vi "Test02_GPU_vs_CPU_Erode.vi"() -> ()   [LabVIEW 2018]
uses:
  <vilib>/vision/NI_Vision_Development_Module.lvlib
  <userlib>/_MGI/1D Array/MGI Average/MGI Average (SGL[]).vi
panel:
  out "Processor History":sgl(graph)
  in  "Stop CPU 2":bool
  out "CPU Average":sgl
  out "error out":errorcluster
  out "CPU Usage (%)":sgl(slide) scale=0.0..100.0
  in  "Time Target (s)":dbl=20.0
  in  "Erode radio":i32=1
  in  "Threshold max":i32=240
  in  "Threshold min":i32=70
  in  "Image Path":path=path "D:/UJI/TFG/TFG_Repositorio/Proyecto/img_to_erode_media.png"
  in  "Start":bool
  in  "Stop GPU":bool
  in  "Stop CPU":bool
  in  "Erode kernel":i32[][](array[numeric])=[[1, 1, 1], [1, 1, 1], [1, 1, 1]]
  out "Image Out CPU":T1(plugin-control)
  out "Image In":T1(plugin-control)
  out "Image Out GPU":T1(plugin-control)
  out "Processed Images":i32
  in  "Threshold range":cluster{"Lower value":sgl, "Upper value":sgl}={"Lower value"=70.0, "Upper value"=240.0} {"Upper value" format="%.2f"; "Lower value" format="%.2f"}
  out "Threhsold Time (ms)":dbl
  out "Erode Time (ms)":dbl
  out "Total Time (ms)":dbl
  out "Error out CPU":errorcluster
  in  "Error in":errorcluster caption="Error in CPU (no error)"
  out "error_cuda_free":i32
  out "error_gpu_to_cpu":i32
  out "error_cpu_to_gpu":i32
  out "Cuda Free Time (ms)":dbl
  out "Set IMG Param Time (ms)":dbl
  out "Total Time (ms)":dbl
  out "Copy to CPU Time (ms)":dbl
  out "Erode Time (ms)":dbl
  out "Threshold Time (ms)":dbl
  out "Copy to GPU Time (ms)":dbl
  out "Processed Images":i32
  out "Error out GPU":errorcluster
  in  "Error":errorcluster caption="Error in GPU (no error)"
  # "GPU CUDA -"
  # "ERODE - GPU vs CPU"
  # "GPU Time Results"
  # "Configuration"
  # "CPU Time Results"
  # "GPU Parameters"
  # "CPU Parameters"
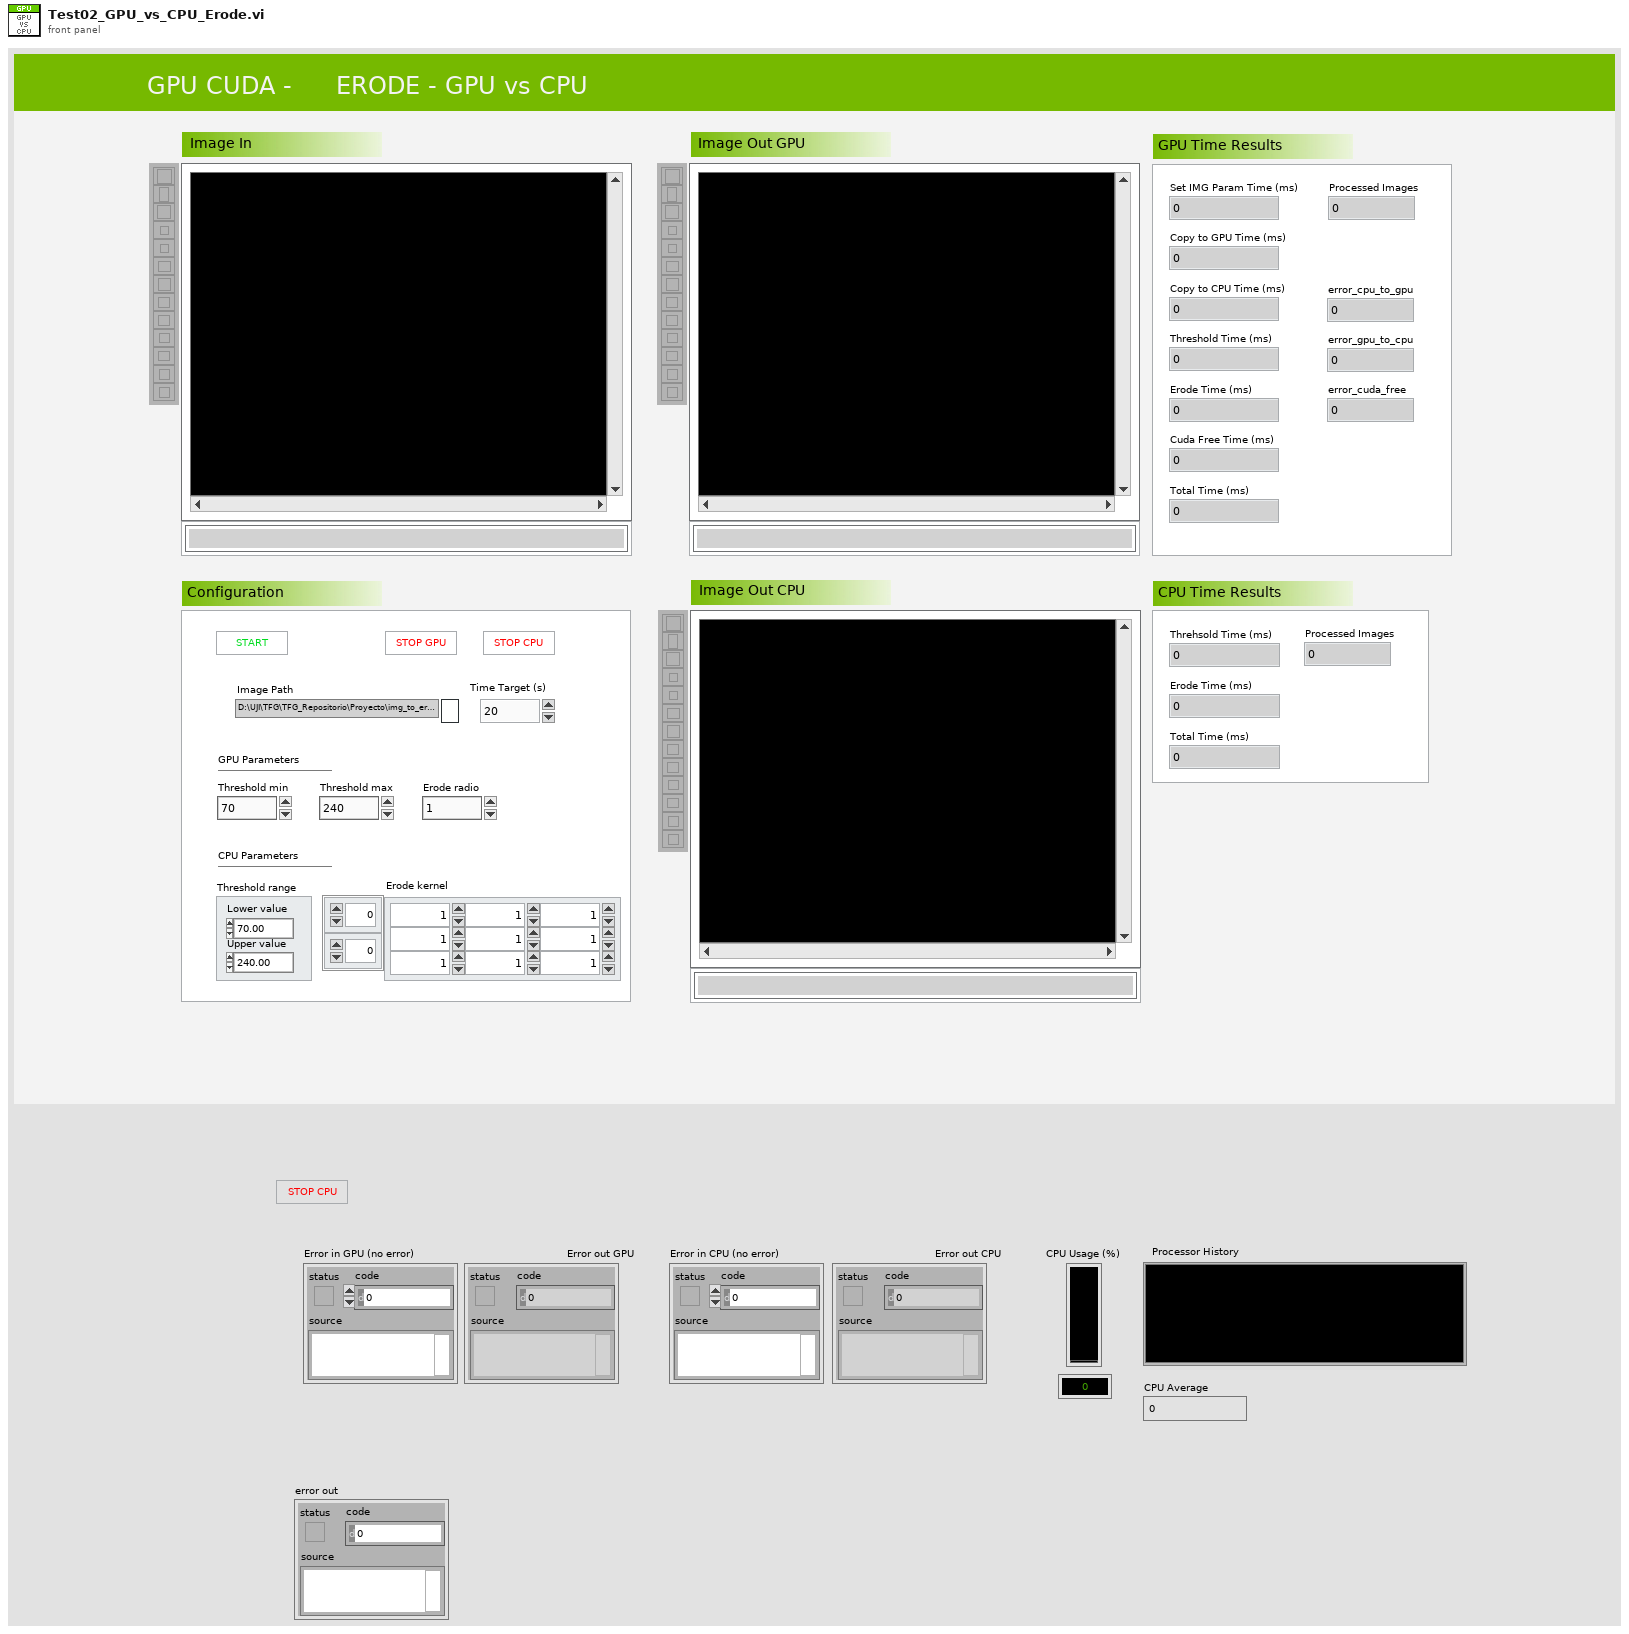
[diagram p1: front panel]
types:
  T1 = typedef "IMAQ Image.ctl" = refnum<image>
  T2 = enum32{"AutoM", "Close", "Dilate", "Erode", "Gradient", "Gradient out", "Gradient in", "Hit miss", "Open", "PClose", "POpen", "Thick", "Thin"}
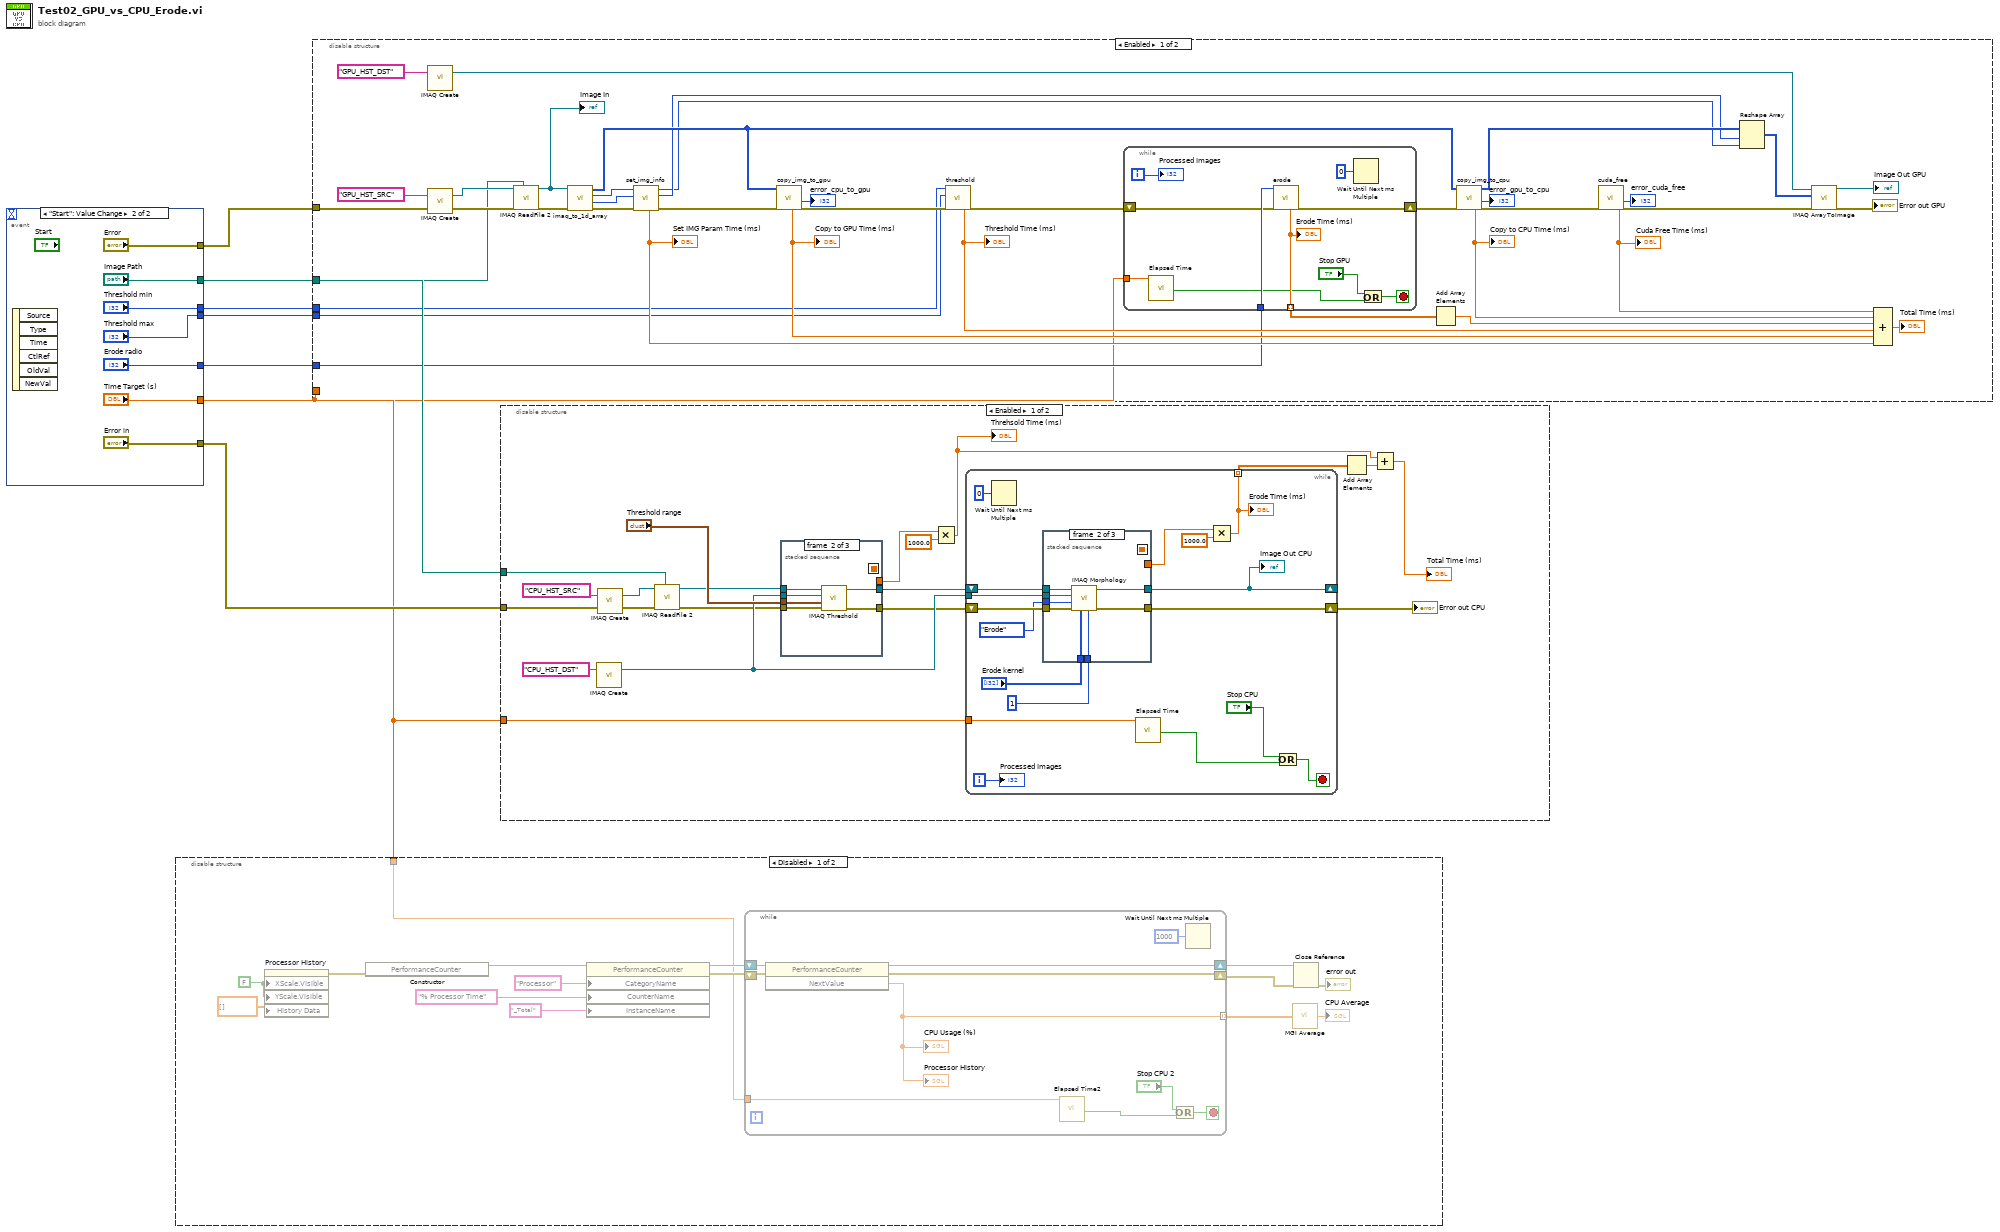
[diagram p0: block diagram]
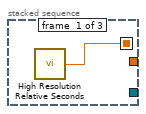
[diagram p4: hidden frame]
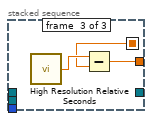
[diagram p5: hidden frame]
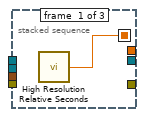
[diagram p6: hidden frame]
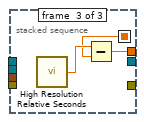
[diagram p7: hidden frame]
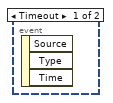
[diagram p9: hidden frame]
diagram:
  n1 = event shown="[1] \"Start\": Value Change" {
    selector: _ -> [_ _]
    dyn-events: _ -> [_ _]
    timeout: _ -> [_ _]
    tunnel: [_ "Error"] -> w7
    tunnel: [_ "Error in"] -> w6
    tunnel: [_ "Erode radio"] -> w5
    tunnel: [_ "Threshold max"] -> w4
    tunnel: [_ "Threshold min"] -> w3
    tunnel: [_ "Time Target (s)"] -> w1
    tunnel: [_ "Image Path"] -> w2
    event Timeout {
      n2 = event-data() -> ()  [unwired: 1 in, 3 out]
    }
    event "Start": Value Change {
      n3 = event-data() -> ()  [unwired: 1 in, 6 out]
    }
  }
  n4 = disable-structure shown="Disabled" {
    disable-tunnel: w1 -> [w18 _]
    frame Disabled {
      w17 = FALSE ("X Scale.Visible")
      n5 = property on="Processor History" class="WFChart (strict)"("XScale.Visible"=w17, "YScale.Visible"=w17, "History Data"=sgl[] []) -> (error out=w15:errorcluster)  [unwired: 2 in, 1 out]
      n6 = constructor class="PerformanceCounter" ("Constructor Node")(error in=w15) -> (reference out=w21:refnum<k24>)  [unwired: 2 in, 2 out]
      n7 = property on="Property Node" class="PerformanceCounter"(reference=w21, "CategoryName"="Processor", "CounterName"="% Processor Time", "InstanceName"="_Total") -> (reference out=w27:refnum<k24>, error out=w26:errorcluster)  [unwired: 1 in]
      n8 = while {
        shift-right: [w36] -> w25
        shift-left: w27 -> [w39]
        shift-right: [w37] -> w22
        shift-left: w26 -> [w38]
        tunnel: [w30] -> w20 mode=indexing
        tunnel: w18 -> [w31]
        stop <- w32 stop-if-true
        n9 = invoke on="Invoke Node" class="PerformanceCounter" method="NextValue"(reference=w39, error in=w38) -> (reference out=w36:refnum<k24>, error out=w37:errorcluster, "NextValue"=w30:sgl)  [unwired: 1 in]
        "CPU Usage (%)" <- w30
        "Processor History" <- w30
        n10 = call "Elapsed Time2"("Time Target (s)"=w31) -> ("Time has Elapsed"=w33:bool)  [unwired: 11 in, 7 out]
        n11 = Or(x="Stop CPU 2", y=w33) -> (x .or. y?=w32:bool)
        n12 = Wait Until Next ms Multiple(millisecond multiple=u32 1000) -> ()  [unwired: 1 out]
      }
      n13 = call-poly <userlib>:"MGI Average.vi"("Single[]"=w20) -> ("Average"=→"CPU Average":sgl)  [unwired: 1 in]
      n14 = Close Reference(reference=w25, error in (no error)=w22) -> (error out=→"error out":errorcluster)
    }
    frame Enabled {
    }
  }
  n15 = disable-structure shown="Enabled" {
    disable-tunnel: w7 -> [w45 _]
    disable-tunnel: w5 -> [w44 _]
    disable-tunnel: w4 -> [w43 _]
    disable-tunnel: w3 -> [w42 _]
    disable-tunnel: w1 -> [w41 _]
    disable-tunnel: w2 -> [w40 _]
    frame Enabled {
      n16 = call "IMAQ Create"("Image Name"="GPU_HST_DST") -> ("New Image"=w76:T1)  [unwired: 4 in, 1 out]
      n17 = call "IMAQ Create"("Image Name"="GPU_HST_SRC", "error in (no error)"=w45) -> ("New Image"=w78:T1, "error out"=w75:errorcluster)  [unwired: 3 in]
      n18 = call "IMAQ ReadFile 2"("File Path"=w40, "error in (no error)"=w75, "Image"=w78) -> ("error out"=w56:errorcluster, "Image Out"=w46:T1)  [unwired: 4 in, 3 out]
      "Image In" <- w46
      n19 = call "imaq_to_1d_array.vi"("Error in"=w56, "Image (in)"=w46) -> ("Error out"=w55:errorcluster, "Height"=w52:i32, "Width"=w53:i32, "Hst Src Image array (out)"=w54:u8[])  [unwired: 6 in]
      n20 = call "set_img_info.vi"("Error in"=w55, "Height (in)"=w52, "Width (in)"=w53) -> ("Error out"=w68:errorcluster, "Height (out)"=w51:i32, "Width (out)"=w50:i32, "Set IMG Parameters Time (ms)"=w67:dbl)  [unwired: 5 in]
      "Set IMG Param Time (ms)" <- w67
      n21 = call "copy_img_to_gpu.vi"("Error in"=w68, "Hst Src Image (in)"=w54) -> ("Error out"=w59:errorcluster, "error_code"=→"error_cpu_to_gpu":i32, "Copy to GPU Time (ms)"=w69:dbl)  [unwired: 6 in, 1 out]
      "Copy to GPU Time (ms)" <- w69
      n22 = call "threshold.vi"("Error in"=w59, "Threshold max (in)"=w43, "Threshold min (in)"=w42) -> ("Error out"=w57:errorcluster, "Threshold Time (ms)"=w60:dbl)  [unwired: 4 in, 3 out]
      "Threshold Time (ms)" <- w60
      n23 = while {
        tunnel: w44 -> [w89]
        tunnel: [w86] -> w49 mode=indexing
        shift-right: [w88] -> w58
        shift-left: w57 -> [w87]
        tunnel: w41 -> [w80]
        i -> [w85]
        stop <- w83 stop-if-true
        n24 = call "Elapsed Time"("Time Target (s)"=w80) -> ("Time has Elapsed"=w82:bool)  [unwired: 11 in, 7 out]
        n25 = call "erode.vi"("Error in"=w87, "Erode Radio (in)"=w89) -> ("Error out"=w88:errorcluster, "Erode Time (ms)"=w86:dbl)  [unwired: 6 in, 2 out]
        "Erode Time (ms)" <- w86
        n26 = Wait Until Next ms Multiple(millisecond multiple=u32 0) -> ()  [unwired: 1 out]
        n27 = Or(x="Stop GPU", y=w82) -> (x .or. y?=w83:bool)
        "Processed Images" <- w85
      }
      n28 = Add Array Elements(numeric array=w49) -> (sum=w48:dbl)
      n29 = call "copy_img_to_cpu.vi"("Error in"=w58, "Hst Dst Image (in)"=w54) -> ("Error out"=w66:errorcluster, "error_code"=→"error_gpu_to_cpu":i32, "Hst Dst Image (out)"=w74:u8[], "Copy to CPU Time (ms)"=w72:dbl)  [unwired: 6 in]
      "Copy to CPU Time (ms)" <- w72
      n30 = call "cuda_free.vi"("Error in"=w66) -> ("Error out"=w65:errorcluster, "error_code"=→"error_cuda_free":i32, "Cuda Free Time (ms)"=w64:dbl)  [unwired: 8 in]
      "Cuda Free Time (ms)" <- w64
      n31 = Reshape Array(w74, w51, w50) -> (w70:u8[][])
      n32 = call "IMAQ ArrayToImage"("error in (no error)"=w65, "Image Pixels (U8)"=w70, "Image"=w76) -> ("error out"=→"Error out GPU":errorcluster, "Image Out"=→"Image Out GPU":T1)  [unwired: 7 in]
      n33 = Compound Arithmetic op=ADD(w64, w72, w48, w60, w69, w67) -> (→"Total Time (ms)":dbl)
    }
    frame Disabled {
    }
  }
  n34 = disable-structure shown="Enabled" {
    disable-tunnel: w6 -> [w92 _]
    disable-tunnel: w1 -> [w91 _]
    disable-tunnel: w2 -> [w90 _]
    frame Enabled {
      n35 = call "IMAQ Create"("Image Name"="CPU_HST_DST") -> ("New Image"=w104:T1)  [unwired: 4 in, 1 out]
      n36 = call "IMAQ Create"("Image Name"="CPU_HST_SRC", "error in (no error)"=w92) -> ("New Image"=w108:T1, "error out"=w109:errorcluster)  [unwired: 3 in]
      n37 = call "IMAQ ReadFile 2"("File Path"=w90, "error in (no error)"=w109, "Image"=w108) -> ("error out"=w103:errorcluster, "Image Out"=w102:T1)  [unwired: 4 in, 3 out]
      n38 = stacked-sequence {
        seq-local: [w139 _ _] -> [_ _ w147]
        tunnel: w103 -> [_ w142 _]
        tunnel: w102 -> [_ w145 _]
        tunnel: "Threshold range" -> [_ w143 _]
        tunnel: w104 -> [_ w144 _]
        tunnel: [_ w141 _] -> w101
        tunnel: [_ w140 _] -> w100
        tunnel: [_ _ w146] -> w97
        frame #0 {
          n39 = call <vilib>:"High Resolution Relative Seconds.vi"() -> ("relative seconds"=w139:dbl)
        }
        frame #1 {
          n40 = call "IMAQ Threshold"("error in (no error)"=w142, "Range"=w143, "Image Dst"=w144, "Image Src"=w145) -> ("error out"=w140:errorcluster, "Image Dst Out"=w141:T1)  [unwired: 6 in]
        }
        frame #2 {
          n41 = call <vilib>:"High Resolution Relative Seconds.vi"() -> ("relative seconds"=w148:dbl)
          n42 = Subtract(x=w148, y=w147) -> (x-y=w146:dbl)
        }
      }
      n43 = Multiply(x=w97, y=1000.0) -> (x*y=w96:dbl)
      "Threhsold Time (ms)" <- w96
      n44 = while {
        tunnel: [w120] -> w94 mode=indexing
        tunnel: w104 -> [w118]
        shift-right: [w113] -> _
        shift-left: w101 -> [w126]
        shift-right: [w119] -> w95
        shift-left: w100 -> [w125]
        tunnel: w91 -> [w110]
        i -> [w114]
        stop <- w116 stop-if-true
        n45 = Wait Until Next ms Multiple(millisecond multiple=u32 0) -> ()  [unwired: 1 out]
        n46 = stacked-sequence {
          seq-local: [w127 _ _] -> [_ _ w137]
          tunnel: w126 -> [_ w135 _]
          tunnel: w118 -> [_ w134 _]
          tunnel: w125 -> [_ w133 _]
          tunnel: [_ w132 _] -> w113
          tunnel: T2."Erode" ("Operation") -> [_ w131 _]
          tunnel: 1 ("Number of iterations (1)") -> [_ w130 _]
          tunnel: [_ _ w136] -> w121
          tunnel: [_ w129 _] -> w119
          tunnel: "Erode kernel" -> [_ w128 _]
          frame #0 {
            n47 = call <vilib>:"High Resolution Relative Seconds.vi"() -> ("relative seconds"=w127:dbl)
          }
          frame #1 {
            n48 = call "IMAQ Morphology"("Number of iterations (1)"=w130, "Structuring Element"=w128, "error in (no error)"=w133, "Operation"=w131, "Image Dst"=w134, "Image Src"=w135) -> ("error out"=w129:errorcluster, "Image Dst Out"=w132:T1)  [unwired: 4 in]
          }
          frame #2 {
            n49 = call <vilib>:"High Resolution Relative Seconds.vi"() -> ("relative seconds"=w138:dbl)
            n50 = Subtract(x=w138, y=w137) -> (x-y=w136:dbl)
          }
        }
        "Image Out CPU" <- w113
        n51 = call "Elapsed Time"("Time Target (s)"=w110) -> ("Time has Elapsed"=w117:bool)  [unwired: 11 in, 7 out]
        n52 = Multiply(x=w121, y=1000.0) -> (x*y=w120:dbl)
        "Erode Time (ms)" <- w120
        n53 = Or(x="Stop CPU", y=w117) -> (x .or. y?=w116:bool)
        "Processed Images" <- w114
      }
      "Error out CPU" <- w95
      n54 = Add Array Elements(numeric array=w94) -> (sum=w93:dbl)
      n55 = Add(x=w96, y=w93) -> (x+y=→"Total Time (ms)":dbl)
    }
    frame Disabled {
    }
  }
